vi "Queue Last Ack.vi"(10 "Queue Actor":refnum<class "Queue Actor.lvclass">, 11 "Base Queue Actor in":refnum<class "Base Queue Actor.lvclass">) -> (3 "Base Queue Actor out":refnum<class "Base Queue Actor.lvclass">)   [LabVIEW 2021, in "jettl.lvlib" / "Base Queue Actor.lvclass"]
uses:
  Base Queue Actor.lvclass
  Queue Actor/Queue Actor.lvclass
  Msg/Msg/Msg.lvclass
  Base Queue Actor.lvclass/Base Queue Actor.ctl
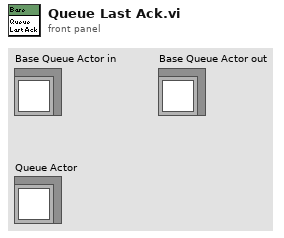
[diagram p1: front panel]
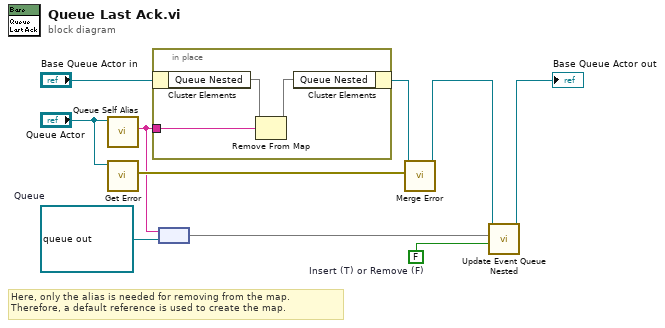
[diagram p0: block diagram]
diagram:
  w1 = refnum<data-value> refnum  # Queue
  w7 = FALSE  # Insert (T) or Remove (F)
  # "Here, only the alias is needed for removing from the map. Therefore, a default reference is used to create the map."
  n1 = call-dynamic "Queue Self Alias.vi"("Actor in"="Queue Actor") -> ("Queue Self Alias"=w3:string)  [unwired: 10 in]
  n2 = call-dynamic "Get Error.vi"("Actor in"="Queue Actor") -> ("Error"=w10:errorcluster)  [unwired: 10 in]
  n3 = in-place {
    in-place-border: w3 -> [w11]
    n4 = in-place-cluster #1("Base Queue Actor in") -> ("Queue Nested"=w12:map{string, refnum<data-value>})
    n5 = Remove From Map(10:w11, 11:w12) -> (3:w13:map{string, refnum<data-value>})  [unwired: 2 out]
    n6 = in-place-cluster #1("Queue Nested"=w13) -> (w9:refnum<class "Base Queue Actor.lvclass">)
  }
  n7 = node(w3, w1) -> (w2:map{string, refnum<data-value>})
  n8 = call-dynamic "Merge Error.vi"("Error"=w10, "Base Queue Actor in"=w9) -> ("Base Queue Actor out"=w6:refnum<class "Base Queue Actor.lvclass">)  [unwired: 9 in]
  n9 = call "Update Event Queue Nested.vi"("Insert (T) or Remove (F)"=w7, "Queue Nested"=w2, "Base Queue Actor in"=w6) -> ("Base Queue Actor out"=→"Base Queue Actor out":refnum<class "Base Queue Actor.lvclass">)  [unwired: 8 in]
